vi "test to be deleted.vi"   [LabVIEW 2016]
types:
  T1 = typedef "CAN Refnum.ctl" = refnum<k1>
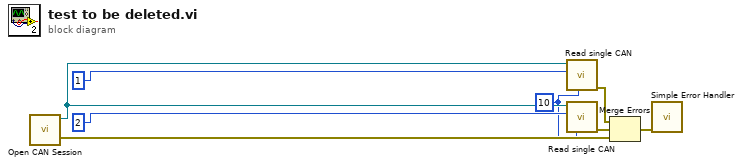
[diagram p0: block diagram]
diagram:
  w1 = 10 ("timeout in ms (-1)")
  n1 = call "Open CAN Session.vi"() -> ("error out"=w3:errorcluster, "CAN Session"=w8:T1)  [unwired: 10 in]
  n2 = call "Read single CAN.vi"("timeout in ms (-1)"=w1, "ID"=1, "CAN Session In"=w8) -> ("error out"=w5:errorcluster)  [unwired: 6 in, 2 out]
  n3 = call "Read single CAN.vi"("timeout in ms (-1)"=w1, "ID"=2, "CAN Session In"=w8) -> ("error out"=w4:errorcluster)  [unwired: 6 in, 2 out]
  n4 = Merge Errors(w5, w4, w3) -> (w2:errorcluster)
  n5 = call <vilib>:"Simple Error Handler.vi"("error in (no error)"=w2) -> ()  [unwired: 4 in, 5 out]
